vi "Focus Stop.vi"(8 "error in (no error)":errorcluster, 10 "Motor (0:n-1)":i32, 11 "ArduinoFocus in":refnum<class "ArduinoFocus.lvclass">) -> (0 "error out":errorcluster, 3 "ArduinoFocus out":refnum<class "ArduinoFocus.lvclass">)   [LabVIEW 2022 SP3, in "ArduinoFocus.lvclass"]
uses:
  ArduinoFocus.lvclass
  ArduinoFocus.lvclass/ArduinoFocus.ctl
  Focus Class/Focus Class.lvclass
  Filter Wheel/Filter Wheel Arduino Control/FW Arduino Control.lvclass
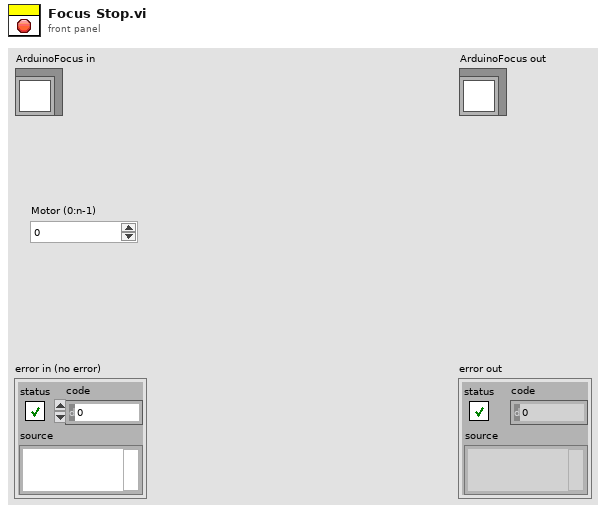
[diagram p1: front panel]
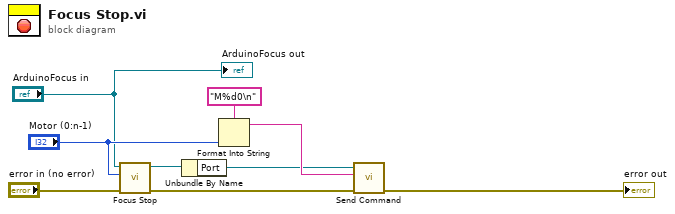
[diagram p0: block diagram]
diagram:
  n1 = call-parent "Focus Stop.vi"("error in (no error)"="error in (no error)", "Motor (0:n-1)"="Motor (0:n-1)", "Focus Class in"="ArduinoFocus in") -> ("error out"=w5:errorcluster, "Focus Class out"=w4:refnum<class "ArduinoFocus.lvclass">)  [unwired: 7 in]
  n2 = Unbundle By Name(w4) -> ("Port"=w3:refnum<visa-resource-name>)
  n3 = Format Into String(format string="M%d0\n", "Motor (0:n-1)") -> (resulting string=w7:string)  [unwired: 2 in, 1 out]
  n4 = call "Send Command.vi"("error in (no error)"=w5, "Command"=w7, "addr"=w3) -> ("error out"=→"error out":errorcluster)  [unwired: 7 in, 1 out]
  "ArduinoFocus out" <- "ArduinoFocus in"
